vi "Get Input DMA Refs.vi"(8 "error in (no error)":errorcluster, 10 "Item GUID":string, 11 "Section Ref in":T1 format="%.0x") -> (0 "error out":errorcluster, 1 "Refs":T2(array[cluster]) {"VS Refs" format="%.0x"}, 2 "DMA Settings":T3[](array[typedef]) {"DMA.Settings"."DMA Host Buffer" items=["1 Second"=1, "2 Seconds"=2, "5 Seconds"=5, "10 Seconds"=10]; "DMA.Settings"."dt" format="%#_p"; "DMA.Settings"."Update Rate" items=["1 Hz"=1, "2 Hz"=2, "5 Hz"=5, "10 Hz"=10]}, 3 "Section Ref out":T1 format="%.0x")   [LabVIEW 2016, in "FPGA Addon System Explorer.lvlib"]
uses:
  FPGA Addon System Explorer.lvlib
  <vilib>/NI Veristand/Custom Device API/Custom Device Item Ref.ctl
  Shared/Compiled.DMASettings.ctl
  Shared/DMA Settings.ctl
  Shared/Delacing Scheme.ctl
  Shared/DMA Acquisition Mode.ctl
  <vilib>/NI Veristand/Custom Device API/Waveform Data Reference.ctl
  Shared/FG Action.ctl
  <vilib>/NI Veristand/Custom Device Tools/Custom Device Utility Library/NI VeriStand - Search for All Items by GUID.vi
  <vilib>/NI Veristand/Custom Device Tools/Custom Device Utility Library/NI VeriStand - Search for Item by GUID.vi
  <vilib>/NI Veristand/Custom Device API/NI VeriStand - Set Item Property.vi
  <vilib>/NI Veristand/Custom Device API/Set Item Property (U32).vi
  <vilib>/NI Veristand/Custom Device API/Set Item Property (Double).vi
  <vilib>/NI Veristand/Custom Device API/Get Item Property (U32).vi
  <vilib>/NI Veristand/Custom Device API/Get Item Property (Double).vi
  Shared/Constants.vi
  <vilib>/NI Veristand/Custom Device API/Get Item Property (String).vi
  Get Host to Target DMAMap.vi
  VeriStand-FPGA-Resource-Manager/Source/find Relative VS Ref.vi
  Get Target to Host DMAMap.vi
  <vilib>/NI Veristand/Custom Device API/NI VeriStand - Get Item Data.vi
  Shared/FPGA Addon Shared.lvlib
  <vilib>/NI VeriStand/Custom Device API/Custom Device API.lvlib
  <vilib>/NI VeriStand/Custom Device Tools/Custom Device Utility Library/Custom Device Utility Library.lvlib
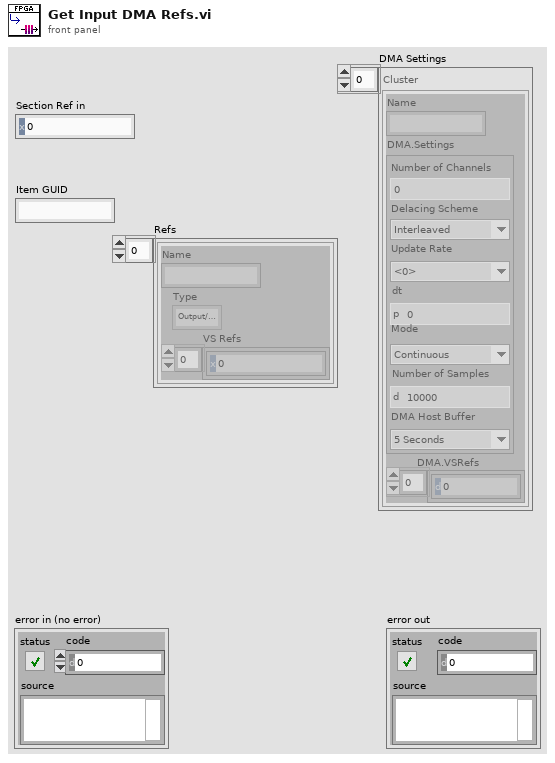
[diagram p1: front panel]
types:
  T1 = typedef "Custom Device API.lvlib/Custom Device Item Ref.ctl" = u64
  T2 = cluster{"Name":string, "Type":enum16{"Output/Write", "Input/Read", "Input/ReadWrite"}, "VS Refs":T1[]}[]
  T3 = typedef "FPGA Addon Shared.lvlib/Compiled.DMASettings.ctl" = cluster{"Name":string, "DMA.Settings":T4, "DMA.VSRefs":T7[]}
  T4 = typedef "FPGA Addon Shared.lvlib/DMA Settings.ctl" = cluster{"Number of Channels":u8, "Delacing Scheme":T5, "Update Rate":u32, "dt":dbl, "Mode":T6, "Number of Samples":u32, "DMA Host Buffer":u32}
  T5 = typedef "FPGA Addon Shared.lvlib/Delacing Scheme.ctl" = enum8{"Interleaved"}
  T6 = typedef "FPGA Addon Shared.lvlib/DMA Acquisition Mode.ctl" = enum8{"Continuous", "Triggered Finite"}
  T7 = typedef "Custom Device API.lvlib/Waveform Data Reference.ctl" = i32
  T8 = typedef "Fifo_DMA_Config.ctl" = cluster{"Name":string, "Depth":u32, "Write? (Deprecated:Use Implementation)":bool, "Physical Channel":u32, "Base Address":u32, "Data Width":u32, "Data Type":T9, "FXP Properties":variant, "Write Window Address":u32, "Implementation":T10, "Control Set":u32}
  T9 = typedef "niFpgaDataTypeControl.ctl" = enum32{"Boolean", "I8", "I16", "I32", "I64", "U8", "U16", "U32", "U64", "FXP", "CustomControl", "SGL"}
  T10 = typedef "niFpgaDmaChannelImplementation.ctl" = enum16{"niFpgaTargetToHost", "niFpgaHostToTarget", "niFpgaPeerToPeerWriter", "niFpgaPeerToPeerReader", "niCoreTargetToHost", "niCoreHostToTarget"}
  T11 = cluster{"Name":string, "Type":enum16{"Output/Write", "Input/Read", "Input/ReadWrite"}, "VS Refs":T1[]}
  T12 = typedef "FPGA Addon Shared.lvlib/FG Action.ctl" = enum8{"GET", "SET"}
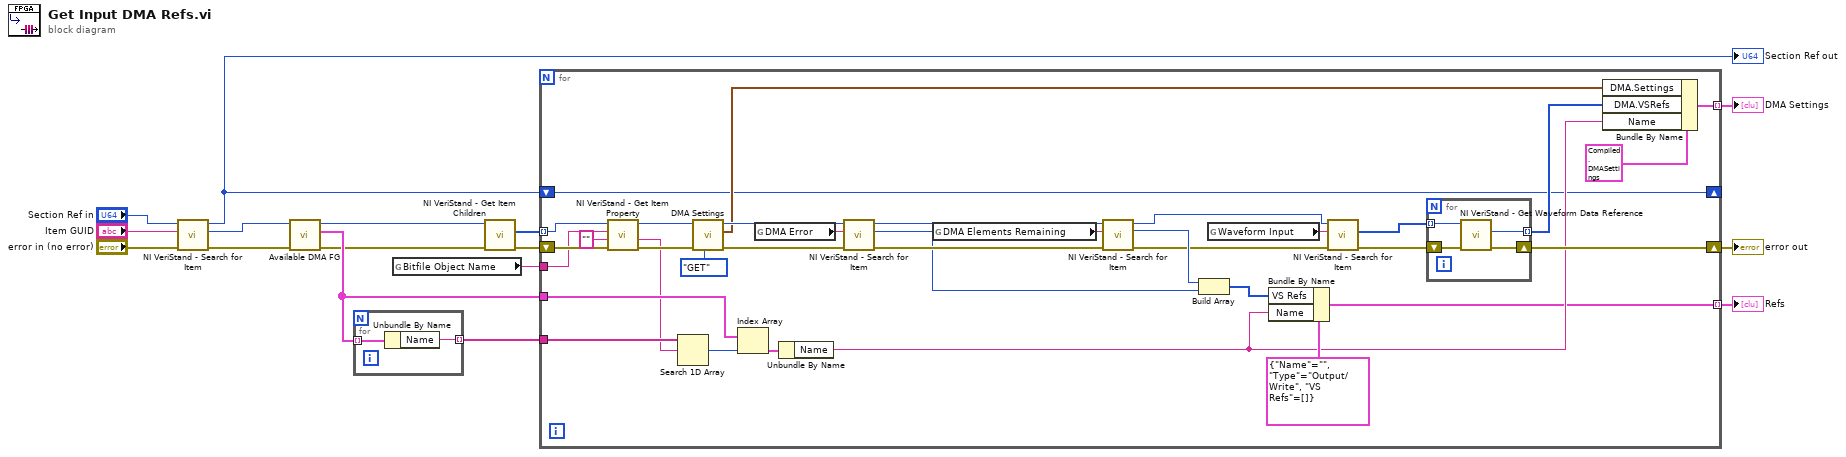
[diagram p0: block diagram]
diagram:
  n1 = call-poly <vilib>:"NI VeriStand - Search for Item.vi"("error in"="error in (no error)", "Item GUID"="Item GUID", "Section Ref in"="Section Ref in") -> ("error out"=w13:errorcluster, "Item Ref"=w15:T1, "Section Ref out"=w2:T1)  [unwired: 5 in, 1 out]
  "Section Ref out" <- w2
  n2 = call "Available DMA FG.vi"("error in (no error)"=w13, "Item Ref"=w15) -> ("error out"=w9:errorcluster, "Available DMA"=w10:T8[], "Item Ref out"=w11:T1)  [unwired: 7 in]
  n3 = for {
    tunnel: w10 -> [w18] mode=indexing
    tunnel: [w17] -> w8 mode=indexing
    n4 = Unbundle By Name(w18) -> ("Name"=w17:string)
  }
  n5 = global read "Constants.vi" "Bitfile Object Name"() -> (w7:string)
  n6 = call <vilib>:"NI VeriStand - Get Item Children.vi"("error in (no error)"=w9, "Item Ref in"=w11) -> ("error out"=w5:errorcluster, "Child Refs"=w6:T1[])  [unwired: 6 in, 2 out]
  n7 = for {
    shift-right: [w26] -> w4
    shift-left: w5 -> [w53]
    tunnel: w6 -> [w52] mode=indexing
    tunnel: w7 -> [w51]
    tunnel: w8 -> [w49]
    tunnel: w10 -> [w48]
    tunnel: [w43] -> w3 mode=indexing
    shift-right: [w19] -> _
    shift-left: w2 -> [w19]
    tunnel: [w21] -> w1 mode=indexing
    n8 = call-poly <vilib>:"NI VeriStand - Get Item Property.vi"("error in (no error)"=w53, "Default Value"="", "Property Name"=w51, "Item Ref in"=w52) -> ("error out"=w42:errorcluster, "Value"=w37:string, "Item Ref out"=w41:T1)  [unwired: 4 in, 1 out]
    n9 = Search 1D Array(1D array=w49, element=w37) -> (index of element=w47:i32)  [unwired: 1 in]
    n10 = call "DMA Settings.vi"("Action"=FG_Action."GET", "error in (no error)"=w42, "Item Ref"=w41) -> ("error out"=w35:errorcluster, "DMA Settings"=w27:T4, "Item Ref out"=w34:T1)  [unwired: 6 in]
    n11 = Index Array(array=w48, index=w47) -> (element=w45:T8)
    n12 = global read "Constants.vi" "DMA Error"() -> (w36:string)
    n13 = Unbundle By Name(w45) -> ("Name"=w23:string)
    n14 = call-poly <vilib>:"NI VeriStand - Search for Item.vi"("error in"=w35, "Item GUID"=w36, "Section Ref in"=w34) -> ("error out"=w32:errorcluster, "Item Ref"=w30:T1, "Section Ref out"=w31:T1)  [unwired: 5 in, 1 out]
    n15 = global read "Constants.vi" "DMA Elements Remaining"() -> (w33:string)
    n16 = call-poly <vilib>:"NI VeriStand - Search for Item.vi"("error in"=w32, "Item GUID"=w33, "Section Ref in"=w31) -> ("error out"=w20:errorcluster, "Item Ref"=w29:T1, "Section Ref out"=w28:T1)  [unwired: 5 in, 1 out]
    n17 = Build Array(w29, w30) -> (w22:T1[])
    n18 = global read "Constants.vi" "Waveform Input"() -> (w38:string)
    n19 = Bundle By Name(cluster=T11 {"Name"="", "Type"=enum."Output/Write", "VS Refs"=[]} ("Group"), "VS Refs"=w22, "Name"=w23) -> (w21:T11)
    n20 = call-poly <vilib>:"NI VeriStand - Search for Item.vi"("error in"=w20, "Item GUID"=w38, "Section Ref in"=w28) -> ("error out"=w40:errorcluster, "Item Refs"=w39:T1[])  [unwired: 5 in, 2 out]
    n21 = for {
      tunnel: w39 -> [w57] mode=indexing
      tunnel: [w56] -> w25 mode=indexing
      shift-right: [w54] -> w26
      shift-left: w40 -> [w55]
      n22 = call <vilib>:"NI VeriStand - Get Waveform Data Reference.vi"("error in (no error)"=w55, "Waveform Ref in"=w57) -> ("error out"=w54:errorcluster, "Waveform Data Reference"=w56:T7)  [unwired: 7 in, 1 out]
    }
    n23 = Bundle By Name(cluster=T3 {"Name"="", "DMA.Settings"={"Number of Channels"=0, "Delacing Scheme"=enum."Interleaved", "Update Rate"=0, "dt"=0.0, "Mode"=enum."Continuous", "Number of Samples"=10000, "DMA Host Buffer"=5}, "DMA.VSRefs"=[]}, "DMA.Settings"=w27, "DMA.VSRefs"=w25, "Name"=w23) -> (w43:T3)
  }
  "error out" <- w4
  "DMA Settings" <- w3
  "Refs" <- w1
